vi "ParseOptions.vi"(8 "error in (no error)":errorcluster, 10 "Options":string[](array[string]), 11 "Test in":refnum<class "Test.lvclass">) -> (0 "error out":errorcluster, 3 "Test out":refnum<class "Test.lvclass">)   [LabVIEW 2014, in "Test.lvclass"]
uses:
  Test.lvclass
  Test.lvclass/Test.ctl
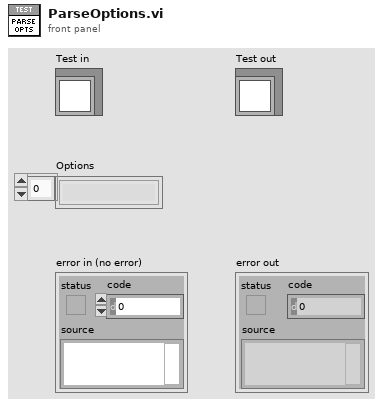
[diagram p1: front panel]
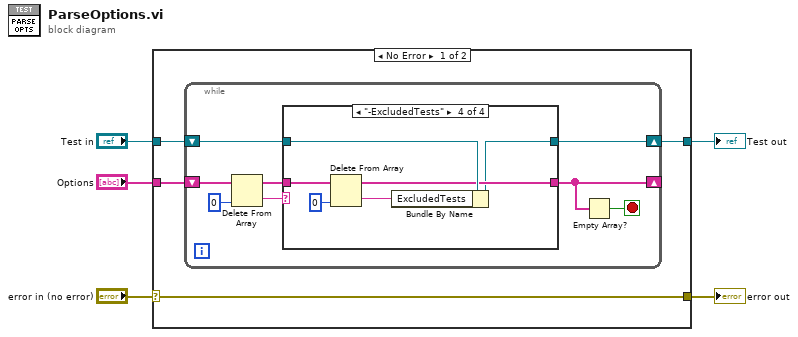
[diagram p0: block diagram]
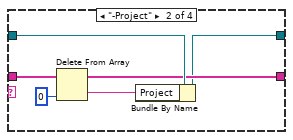
[diagram p3: hidden frame]
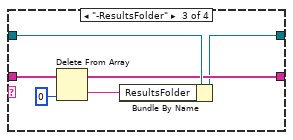
[diagram p4: hidden frame]
diagram:
  n1 = case shown="No Error" "error in (no error)" {
    selector: "error in (no error)" -> [w9 w39]
    tunnel: [w9 w39] -> w1
    tunnel: [w7 w38] -> w4
    tunnel: "Test in" -> [w6 w38]
    tunnel: "Options" -> [w8 _]
    frame No Error {
      n2 = while {
        shift-right: [w13] -> _
        shift-left: w8 -> [w17]
        shift-right: [w11] -> w7
        shift-left: w6 -> [w10]
        stop <- w12 stop-if-true
        n3 = Delete From Array(array=w17, index=0) -> (deleted portion=w15:string, array with subset deleted=w14:string[])  [unwired: 1 in]
        n4 = case shown="\"-ExcludedTests\"" w15 {
          tunnel: [w19 w23 w29 w35] -> w13
          tunnel: w14 -> [w19 w24 w30 w36]
          tunnel: [w18 w21 w27 w33] -> w11
          tunnel: w10 -> [w18 w25 w31 w37]
          frame Default {
          }
          frame "-Project" {
            n5 = Delete From Array(array=w24, index=0) -> (deleted portion=w20:string, array with subset deleted=w23:string[])  [unwired: 1 in]
            n6 = Bundle By Name(cluster=w25, "Project"=w20) -> (w21:refnum<class "Test.lvclass">)
          }
          frame "-ResultsFolder" {
            n7 = Delete From Array(array=w30, index=0) -> (deleted portion=w26:string, array with subset deleted=w29:string[])  [unwired: 1 in]
            n8 = Bundle By Name(cluster=w31, "ResultsFolder"=w26) -> (w27:refnum<class "Test.lvclass">)
          }
          frame "-ExcludedTests" {
            n9 = Delete From Array(array=w36, index=0) -> (deleted portion=w32:string, array with subset deleted=w35:string[])  [unwired: 1 in]
            n10 = Bundle By Name(cluster=w37, "ExcludedTests"=w32) -> (w33:refnum<class "Test.lvclass">)
          }
        }
        n11 = Empty Array?(array=w13) -> (empty?=w12:bool)
      }
    }
    frame Error {
    }
  }
  "error out" <- w1
  "Test out" <- w4
